vi "Detector Log.vi"(8 "error in (no error)":errorcluster, 10 "Log Path":path, 11 "Rows to Add":string[](array[string])) -> (0 "error out":errorcluster)   [LabVIEW 2021]
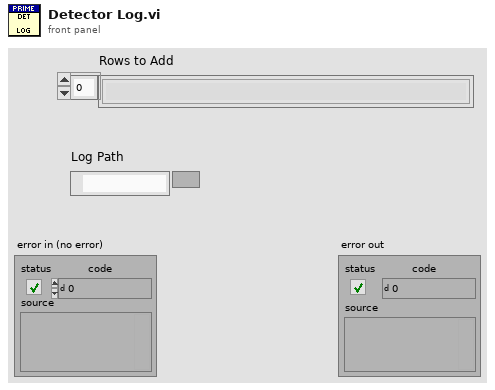
[diagram p1: front panel]
types:
  T1 = enum16{"open", "replace", "create", "open or create", "replace or create", "replace or create with confirmation"}
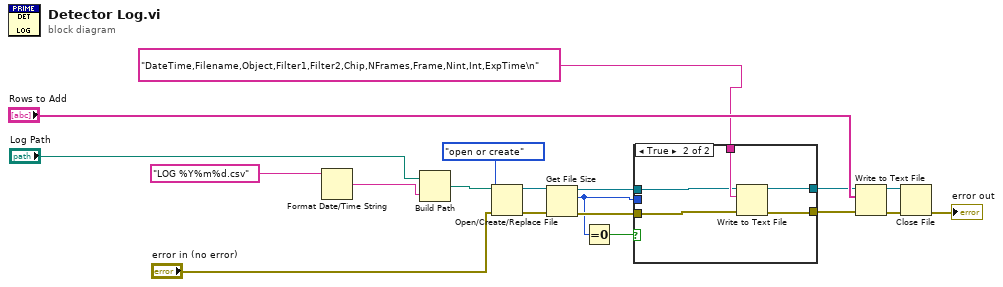
[diagram p0: block diagram]
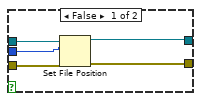
[diagram p2: hidden frame]
diagram:
  n1 = Format Date/Time String(time format string (%c)="LOG %Y%m%d.csv") -> (date/time string=w14:string)  [unwired: 2 in]
  n2 = Build Path(base path="Log Path", name or relative path=w14) -> (appended path=w13:path)
  n3 = Open/Create/Replace File(file path (use dialog)=w13, error in="error in (no error)", operation (0:open)=T1."open or create") -> (refnum out=w11:refnum<file>, error out=w8:errorcluster)  [unwired: 3 in, 1 out]
  n4 = Get File Size(file=w11, error in=w8) -> (refnum out=w10:refnum<file>, size (in bytes)=w6:i64, 0:w9:errorcluster)
  n5 = Equal To 0?(x=w6) -> (x = 0?=w7:bool)
  n6 = case shown="True" w7 {
    tunnel: [w22 w29] -> w16
    tunnel: "DateTime,Filename,Object,Filter1,Filter2,Chip,NFrames,Frame,Nint,Int,ExpTime\n" ("time format string (%c)") -> [_ w28]
    tunnel: w10 -> [w23 w27]
    tunnel: w9 -> [w24 w26]
    tunnel: w6 -> [w21 _]
    tunnel: [w20 w25] -> w3
    frame False {
      n7 = Set File Position(offset (in bytes) (0)=w21, refnum=w23, error in=w24) -> (refnum out=w22:refnum<file>, error out=w20:errorcluster)  [unwired: 1 in]
    }
    frame True {
      n8 = Write to Text File(file (use dialog)=w27, text=w28, error in=w26) -> (refnum out=w29:refnum<file>, error out=w25:errorcluster)  [unwired: 1 in, 1 out]
    }
  }
  n9 = Write to Text File(file (use dialog)=w16, text="Rows to Add", error in=w3) -> (refnum out=w4:refnum<file>, error out=w5:errorcluster)  [unwired: 1 in, 1 out]
  n10 = Close File(refnum=w4, error in=w5) -> (error out=→"error out":errorcluster)  [unwired: 1 out]
